vi "Get flattened data.vi"(8 "error in (no error)":errorcluster, 11 "String D Element in":refnum<class "String D Element.lvclass">) -> (0 "error out":errorcluster, 2 "Flattened data":u8[](array[numeric]), 3 "String D Element out":refnum<class "String D Element.lvclass">)   [LabVIEW 2018, in "D Datagrid Library.lvlib" / "String D Element.lvclass"]
uses:
  String D Element.lvclass
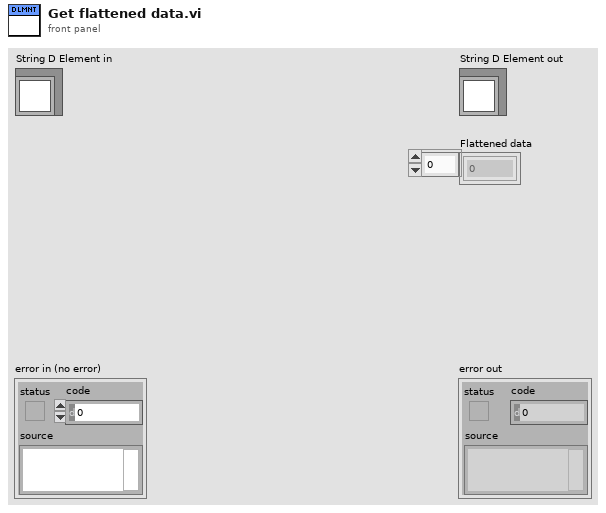
[diagram p1: front panel]
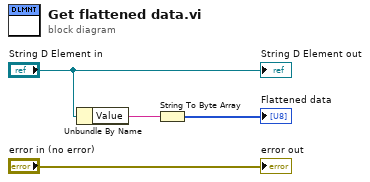
[diagram p0: block diagram]
diagram:
  n1 = Unbundle By Name("String D Element in") -> ("Value"=w2:string)
  n2 = String To Byte Array(string=w2) -> (unsigned byte array=→"Flattened data":u8[])
  "error out" <- "error in (no error)"
  "String D Element out" <- "String D Element in"
